vi "Round 2.vi"(8 "error in (no error)":errorcluster, 11 "KNR in":T1) -> (0 "error out":errorcluster, 3 "KNR out":T1)   [LabVIEW 2013]
uses:
  <userlib>/KNR OS 3.0 LabVIEW Toolkit/Type Definition/KNR3 Reference.ctl
  <userlib>/_FPGA Interface Advanced Tools/FPGA Interface Base/FPGA Interface Base.lvclass
  <userlib>/KNR OS 3.0 LabVIEW Toolkit/Type Definition/Resource.ctl
  <userlib>/KNR OS 3.0 LabVIEW Toolkit/Type Definition/DC Motor Port.ctl
  Global 1.vi
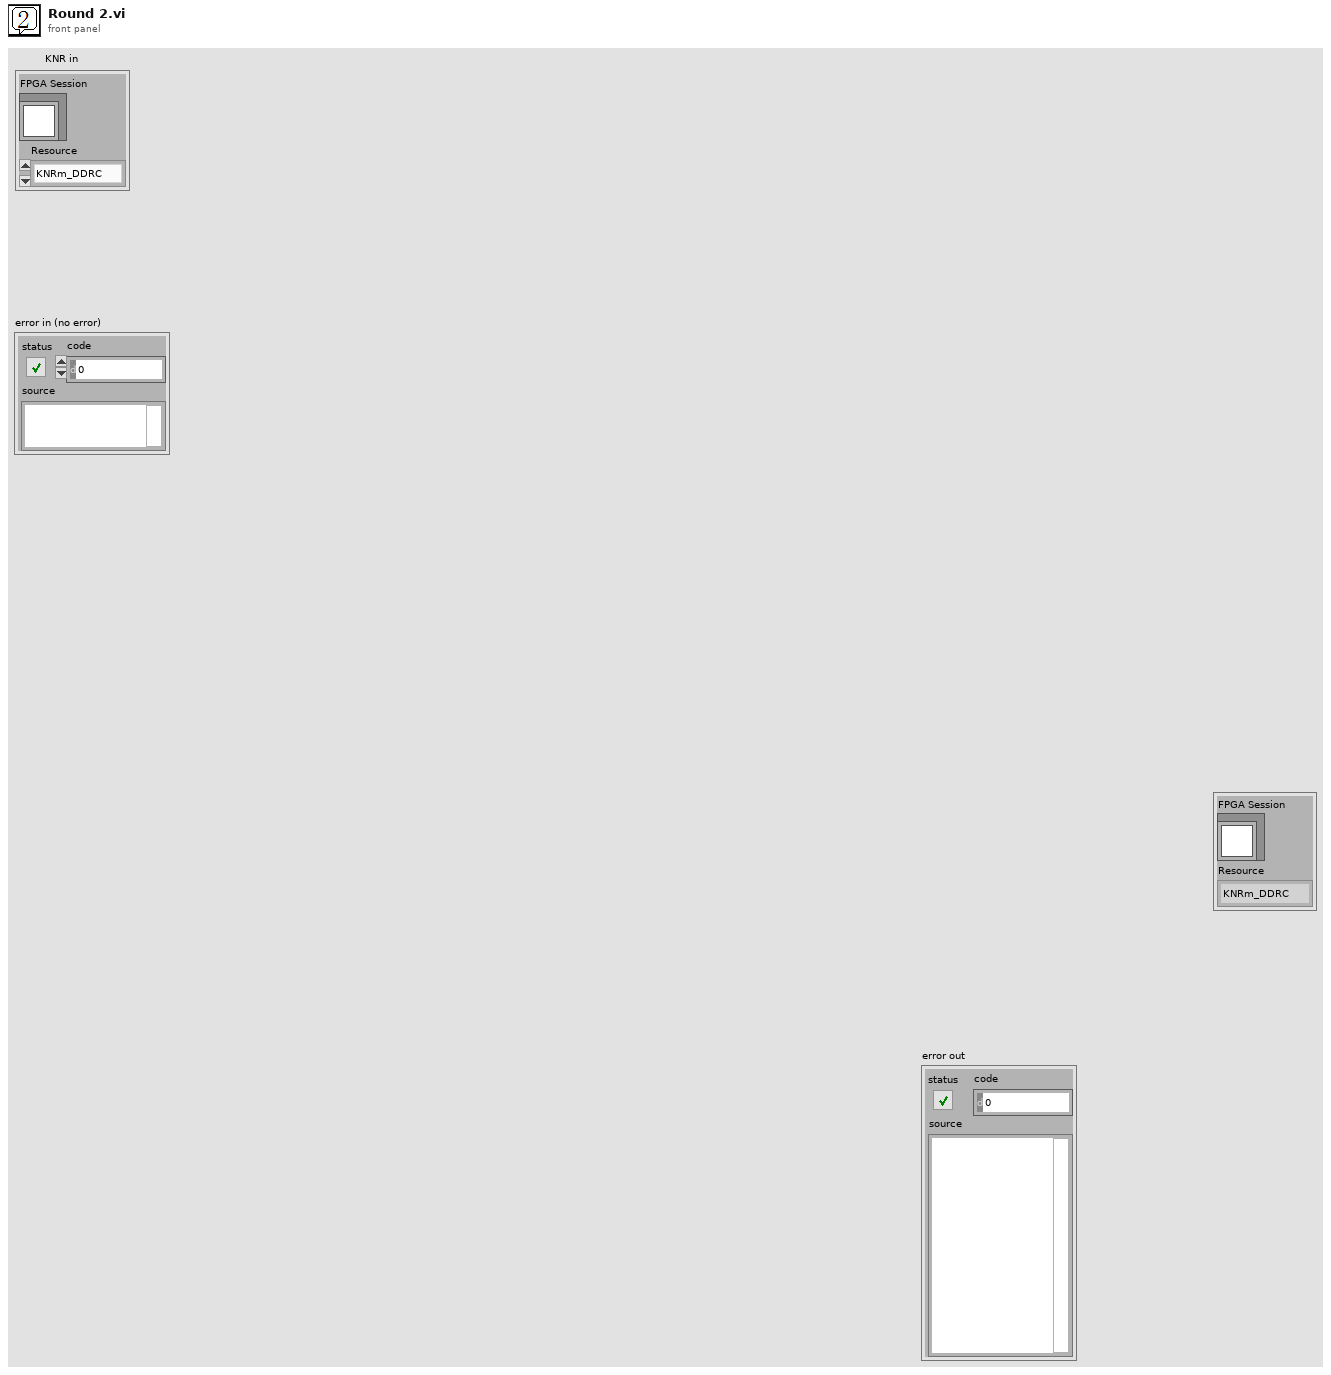
[diagram p1: front panel]
types:
  T1 = typedef "KNR3 Reference.ctl" = cluster{"FPGA Session":refnum<class "FPGA Interface Base.lvclass">, "Resource":T2}
  T2 = typedef "Resource.ctl" = enum16{"KNRm_DDRC", "KNRm_DDDD", "KNRm_DDDR", "KNRm_DDDC", "KNR"}
  T3 = typedef "DC Motor Port.ctl" = u16
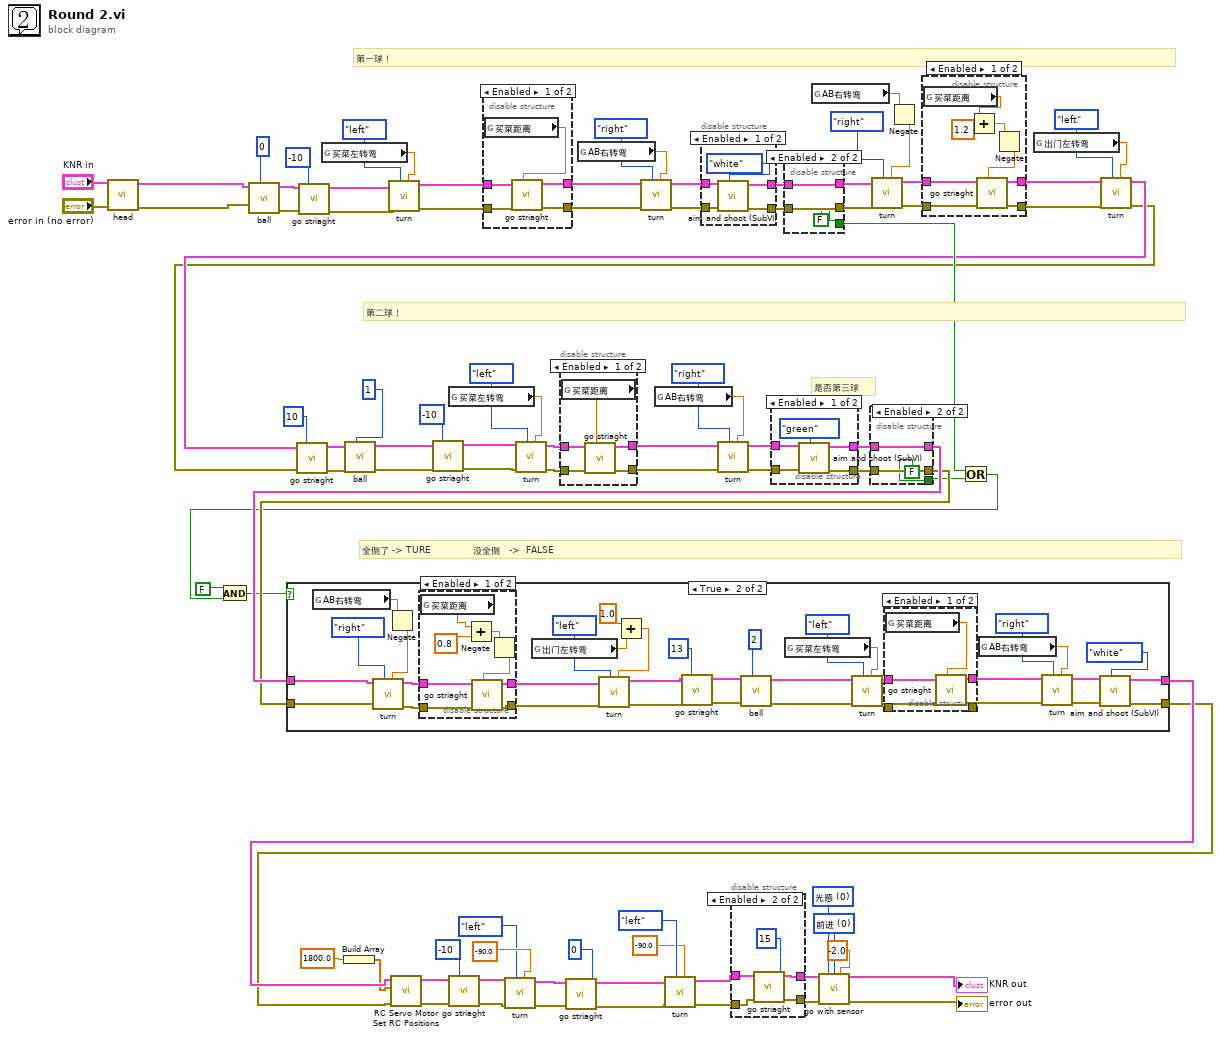
[diagram p0: block diagram]
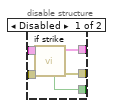
[diagram p2: hidden frame]
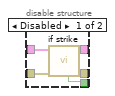
[diagram p3: hidden frame]
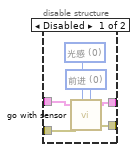
[diagram p4: hidden frame]
diagram:
  w26 = T3 0 items=["前进", "后退"] ("方向")
  w27 = T3 0 items=["光感", "超声波"] ("传感器类型")
  # "是否第三球"
  # "全倒了 -> TURE              没全倒   ->  FALSE"
  # "第二球！"
  # "第一球！"
  n1 = call "head.vi"("error in (no error)"="error in (no error)", "KNR in"="KNR in") -> ("error out"=w1:errorcluster, "KNR out"=w2:T1)  [unwired: 8 in]
  n2 = call "ball.vi"("Numeric"=0, "error in (no error)"=w1, "KNR in"=w2) -> ("error out"=w41:errorcluster, "KNR out"=w42:T1)  [unwired: 6 in, 1 out]
  n3 = call "go striaght.vi"("距离"=-10, "error in (no error)"=w41, "KNR in"=w42) -> ("error out"=w39:errorcluster, "KNR out"=w40:T1)  [unwired: 7 in]
  n4 = global read "Global 1.vi" "买菜左转弯"() -> (w86:dbl)
  n5 = Build Array(1800.0 ("element")) -> (w56:dbl[])
  n6 = call "turn.vi"("Angle"=w86, "side"=enum16{"right", "left"}."left", "error in (no error)"=w39, "KNR in"=w40) -> ("error out"=w87:errorcluster, "KNR out"=w88:T1)  [unwired: 6 in]
  n7 = global read "Global 1.vi" "买菜左转弯"() -> (w69:dbl)
  n8 = disable-structure shown="Enabled" {
    disable-tunnel: w88 -> [w95 w97]
    disable-tunnel: w87 -> [w94 w96]
    disable-tunnel: [w92 w97] -> w83
    disable-tunnel: [w91 w96] -> w82
    frame Enabled {
      n9 = global read "Global 1.vi" "买菜距离"() -> (w93:dbl)
      n10 = call "go striaght.vi"("距离"=w93, "error in (no error)"=w94, "KNR in"=w95) -> ("error out"=w91:errorcluster, "KNR out"=w92:T1)  [unwired: 7 in]
    }
    frame Disabled {
    }
  }
  n11 = global read "Global 1.vi" "AB右转弯"() -> (w85:dbl)
  n12 = call "turn.vi"("Angle"=w85, "side"=enum16{"right", "left"}."right", "error in (no error)"=w82, "KNR in"=w83) -> ("error out"=w49:errorcluster, "KNR out"=w45:T1)  [unwired: 6 in]
  n13 = global read "Global 1.vi" "AB右转弯"() -> (w68:dbl)
  n14 = disable-structure shown="Enabled" {
    disable-tunnel: [w102 w103] -> w54
    disable-tunnel: w49 -> [w101 w103]
    disable-tunnel: w45 -> [w100 w104]
    disable-tunnel: [w99 w104] -> w44
    frame Enabled {
      n15 = call "aim and shoot (SubVI).vi"("pin"=enum16{"white", "green"}."white", "error in (no error)"=w101, "KNR in"=w100) -> ("error out"=w102:errorcluster, "KNR out"=w99:T1)  [unwired: 7 in]
    }
    frame Disabled {
    }
  }
  n16 = disable-structure shown="Enabled" {
    disable-tunnel: w54 -> [w109 w111]
    disable-tunnel: [w108 FALSE] -> w53
    disable-tunnel: [w107 w112] -> w51
    disable-tunnel: [w106 w111] -> w50
    disable-tunnel: w44 -> [w105 w112]
    frame Disabled {
      n17 = call "if strike.vi"("error in (no error)"=w109, "KNR in"=w105) -> ("error out"=w106:errorcluster, "KNR out"=w107:T1, "is strike?"=w108:bool)  [unwired: 7 in]
    }
    frame Enabled {
    }
  }
  n18 = global read "Global 1.vi" "AB右转弯"() -> (w81:dbl)
  n19 = Negate(x=w81) -> (-x=w79:dbl)
  n20 = call "turn.vi"("Angle"=w79, "side"=enum16{"right", "left"}."right", "error in (no error)"=w50, "KNR in"=w51) -> ("error out"=w77:errorcluster, "KNR out"=w78:T1)  [unwired: 6 in]
  n21 = disable-structure shown="Enabled" {
    disable-tunnel: w78 -> [w120 w122]
    disable-tunnel: w77 -> [w119 w121]
    disable-tunnel: [w117 w122] -> w75
    disable-tunnel: [w116 w121] -> w74
    frame Enabled {
      n22 = global read "Global 1.vi" "买菜距离"() -> (w114:dbl)
      n23 = Add(x=w114, y=1.2) -> (x+y=w113:dbl)
      n24 = Negate(x=w113) -> (-x=w118:dbl)
      n25 = call "go striaght.vi"("距离"=w118, "error in (no error)"=w119, "KNR in"=w120) -> ("error out"=w116:errorcluster, "KNR out"=w117:T1)  [unwired: 7 in]
    }
    frame Disabled {
    }
  }
  n26 = global read "Global 1.vi" "出门左转弯"() -> (w46:dbl)
  n27 = call "turn.vi"("Angle"=w46, "side"=enum16{"right", "left"}."left", "error in (no error)"=w74, "KNR in"=w75) -> ("error out"=w7:errorcluster, "KNR out"=w8:T1)  [unwired: 6 in]
  n28 = call "go striaght.vi"("距离"=10, "error in (no error)"=w7, "KNR in"=w8) -> ("error out"=w36:errorcluster, "KNR out"=w37:T1)  [unwired: 7 in]
  n29 = call "ball.vi"("Numeric"=1, "error in (no error)"=w36, "KNR in"=w37) -> ("error out"=w32:errorcluster, "KNR out"=w34:T1)  [unwired: 6 in, 1 out]
  n30 = call "go striaght.vi"("距离"=-10, "error in (no error)"=w32, "KNR in"=w34) -> ("error out"=w31:errorcluster, "KNR out"=w33:T1)  [unwired: 7 in]
  n31 = call "turn.vi"("Angle"=w69, "side"=enum16{"right", "left"}."left", "error in (no error)"=w31, "KNR in"=w33) -> ("error out"=w70:errorcluster, "KNR out"=w71:T1)  [unwired: 6 in]
  n32 = disable-structure shown="Enabled" {
    disable-tunnel: w71 -> [w127 w129]
    disable-tunnel: w70 -> [w126 w128]
    disable-tunnel: [w124 w129] -> w66
    disable-tunnel: [w123 w128] -> w65
    frame Enabled {
      n33 = global read "Global 1.vi" "买菜距离"() -> (w125:dbl)
      n34 = call "go striaght.vi"("距离"=w125, "error in (no error)"=w126, "KNR in"=w127) -> ("error out"=w123:errorcluster, "KNR out"=w124:T1)  [unwired: 7 in]
    }
    frame Disabled {
    }
  }
  n35 = call "turn.vi"("Angle"=w68, "side"=enum16{"right", "left"}."right", "error in (no error)"=w65, "KNR in"=w66) -> ("error out"=w47:errorcluster, "KNR out"=w48:T1)  [unwired: 6 in]
  n36 = disable-structure shown="Enabled" {
    disable-tunnel: [w133 w136] -> w64
    disable-tunnel: [w134 w135] -> w63
    disable-tunnel: w48 -> [w132 w136]
    disable-tunnel: w47 -> [w131 w135]
    frame Enabled {
      n37 = call "aim and shoot (SubVI).vi"("pin"=enum16{"white", "green", "left", "right"}."green", "error in (no error)"=w131, "KNR in"=w132) -> ("error out"=w134:errorcluster, "KNR out"=w133:T1)  [unwired: 7 in]
    }
    frame Disabled {
    }
  }
  n38 = disable-structure shown="Enabled" {
    disable-tunnel: w64 -> [w141 w144]
    disable-tunnel: w63 -> [w140 w143]
    disable-tunnel: [w139 w144] -> w62
    disable-tunnel: [w138 w143] -> w61
    disable-tunnel: [w137 FALSE] -> w52
    frame Disabled {
      n39 = call "if strike.vi"("error in (no error)"=w140, "KNR in"=w141) -> ("error out"=w138:errorcluster, "KNR out"=w139:T1, "is strike?"=w137:bool)  [unwired: 7 in]
    }
    frame Enabled {
    }
  }
  n40 = Or(x=w53, y=w52) -> (x .or. y?=w28:bool)
  n41 = And(x=FALSE, y=w28) -> (x .and. y?=w29:bool)
  n42 = case shown="True" w29 {
    tunnel: w62 -> [w146 w161]
    tunnel: w61 -> [w145 w160]
    tunnel: [w146 w163] -> w58
    tunnel: [w145 w162] -> w57
    frame False {
    }
    frame True {
      n43 = global read "Global 1.vi" "AB右转弯"() -> (w180:dbl)
      n44 = Negate(x=w180) -> (-x=w178:dbl)
      n45 = call "turn.vi"("Angle"=w178, "side"=enum16{"right", "left"}."right", "error in (no error)"=w160, "KNR in"=w161) -> ("error out"=w176:errorcluster, "KNR out"=w177:T1)  [unwired: 6 in]
      n46 = disable-structure shown="Enabled" {
        disable-tunnel: w177 -> [w195 w196]
        disable-tunnel: w176 -> [w194 w197]
        disable-tunnel: [_ w196] -> _
        disable-tunnel: [w192 w197] -> w175
        disable-tunnel: [w188 w196] -> w147
        frame Enabled {
          n47 = global read "Global 1.vi" "买菜距离"() -> (w190:dbl)
          n48 = Add(x=w190, y=0.8) -> (x+y=w189:dbl)
          n49 = Negate(x=w189) -> (-x=w193:dbl)
          n50 = call "go striaght.vi"("距离"=w193, "error in (no error)"=w194, "KNR in"=w195) -> ("error out"=w192:errorcluster, "KNR out"=w188:T1)  [unwired: 7 in]
        }
        frame Disabled {
        }
      }
      n51 = global read "Global 1.vi" "出门左转弯"() -> (w156:dbl)
      n52 = Add(x=1.0, y=w156) -> (x+y=w154:dbl)
      n53 = call "turn.vi"("Angle"=w154, "side"=enum16{"right", "left"}."left", "error in (no error)"=w175, "KNR in"=w147) -> ("error out"=w148:errorcluster, "KNR out"=w149:T1)  [unwired: 6 in]
      n54 = call "go striaght.vi"("距离"=13, "error in (no error)"=w148, "KNR in"=w149) -> ("error out"=w150:errorcluster, "KNR out"=w151:T1)  [unwired: 7 in]
      n55 = call "ball.vi"("Numeric"=2, "error in (no error)"=w150, "KNR in"=w151) -> ("error out"=w171:errorcluster, "KNR out"=w172:T1)  [unwired: 6 in, 1 out]
      n56 = global read "Global 1.vi" "买菜左转弯"() -> (w168:dbl)
      n57 = call "turn.vi"("Angle"=w168, "side"=enum16{"right", "left"}."left", "error in (no error)"=w171, "KNR in"=w172) -> ("error out"=w169:errorcluster, "KNR out"=w170:T1)  [unwired: 6 in]
      n58 = disable-structure shown="Enabled" {
        disable-tunnel: w170 -> [w185 w187]
        disable-tunnel: w169 -> [w184 w186]
        disable-tunnel: [w182 w187] -> w165
        disable-tunnel: [w181 w186] -> w164
        frame Enabled {
          n59 = global read "Global 1.vi" "买菜距离"() -> (w183:dbl)
          n60 = call "go striaght.vi"("距离"=w183, "error in (no error)"=w184, "KNR in"=w185) -> ("error out"=w181:errorcluster, "KNR out"=w182:T1)  [unwired: 7 in]
        }
        frame Disabled {
        }
      }
      n61 = global read "Global 1.vi" "AB右转弯"() -> (w167:dbl)
      n62 = call "turn.vi"("Angle"=w167, "side"=enum16{"right", "left"}."right", "error in (no error)"=w164, "KNR in"=w165) -> ("error out"=w158:errorcluster, "KNR out"=w159:T1)  [unwired: 6 in]
      n63 = call "aim and shoot (SubVI).vi"("pin"=enum16{"white", "green"}."white", "error in (no error)"=w158, "KNR in"=w159) -> ("error out"=w162:errorcluster, "KNR out"=w163:T1)  [unwired: 7 in]
    }
  }
  n64 = call <userlib>:"RC Servo Motor Set RC Positions.vi"("error in (no error)"=w57, "RC Pulse Width (1500 uS)"=w56, "KNR in"=w58) -> ("error out"=w18:errorcluster, "KNR out"=w19:T1)  [unwired: 7 in]
  n65 = call "go striaght.vi"("距离"=-10, "error in (no error)"=w18, "KNR in"=w19) -> ("error out"=w20:errorcluster, "KNR out"=w21:T1)  [unwired: 7 in]
  n66 = call "turn.vi"("Angle"=-90.0, "side"=enum16{"right", "left"}."left", "error in (no error)"=w20, "KNR in"=w21) -> ("error out"=w15:errorcluster, "KNR out"=w16:T1)  [unwired: 6 in]
  n67 = call "go striaght.vi"("距离"=0, "error in (no error)"=w15, "KNR in"=w16) -> ("error out"=w11:errorcluster, "KNR out"=w12:T1)  [unwired: 7 in]
  n68 = call "turn.vi"("Angle"=-90.0, "side"=enum16{"right", "left"}."left", "error in (no error)"=w11, "KNR in"=w12) -> ("error out"=w9:errorcluster, "KNR out"=w10:T1)  [unwired: 6 in]
  n69 = disable-structure shown="Enabled" {
    disable-tunnel: [w201 w207] -> w24
    disable-tunnel: [w200 w206] -> w23
    disable-tunnel: w10 -> [w199 w205]
    disable-tunnel: w9 -> [w198 w204]
    frame Disabled {
      w202 = T3 0 items=["前进", "后退"] ("方向")
      w203 = T3 0 items=["光感", "超声波"] ("传感器类型")
      n70 = call "go with sensor.vi"("KNR in"=w199, "传感器类型"=w203, "error in (no error)"=w198, "方向"=w202) -> ("KNR out"=w201:T1, "error out"=w200:errorcluster)  [unwired: 3 in, 1 out]
    }
    frame Enabled {
      n71 = call "go striaght.vi"("距离"=15, "error in (no error)"=w204, "KNR in"=w205) -> ("error out"=w206:errorcluster, "KNR out"=w207:T1)  [unwired: 7 in]
    }
  }
  n72 = call "go with sensor.vi"("KNR in"=w24, "传感器类型"=w27, "方向"=w26, "then go:"=-2.0, "error in (no error)"=w23) -> ("KNR out"=→"KNR out":T1, "error out"=→"error out":errorcluster)  [unwired: 8 in, 1 out]
